vi "caluculate_phase_diff.vi"() -> ()   [LabVIEW 2014]
uses:
  <vilib>/Analysis/3filter.llb/Filter Passband Type.ctl
  <vilib>/addons/Digital Filter Design/_Objects.llb/DFD Quantization Settings.ctl
  <vilib>/addons/Digital Filter Design/_Objects.llb/DFD Quantization Sources.ctl
  <vilib>/measure/matone.llb/Extract Single Tone Information 1 Chan.vi
  <vilib>/Analysis/3filter.llb/IIR Filter (DBL).vi
  <vilib>/addons/Digital Filter Design/Process.llb/DFD Filtering (Array).vi
  <vilib>/addons/Digital Filter Design/FXPLib.llb/DFD FXP to I16 (scalar).vi
  <vilib>/Waveform/WDTOps.llb/WDT Get Waveform Subset DBL.vi
  <vilib>/addons/Digital Filter Design/FXPModel.llb/DFD FXP Quantize Coef (Easy).vi
  <vilib>/addons/Digital Filter Design/CodeGen.llb/DFD FXP C Code Generator.vi
  <vilib>/Utility/VariantDataType/GetNumericFxpInfo.vi
  <vilib>/addons/Digital Filter Design/FXPSim.llb/dfd_Check Input FXP Settings.vi
  <vilib>/addons/Digital Filter Design/FXPSim.llb/dfd_Check SRate Simulation Integer Input.vi
  <vilib>/addons/Digital Filter Design/FXPSim.llb/dfd_FXP Simu.vi
  <vilib>/addons/Digital Filter Design/FXPLib.llb/DFD I16 to FXP (scalar).vi
  <vilib>/addons/Digital Filter Design/_Objects.llb/DFD FXP Statistics Data.ctl
  <vilib>/addons/Digital Filter Design/FXPSim.llb/SimXnode/DFD FXP Simulation.xnode
  <vilib>/addons/Digital Filter Design/_Objects.llb/DFD Filter Obj.ctl
  <vilib>/addons/Digital Filter Design/_Objects.llb/DFD Filter Coef.ctl
  <vilib>/addons/Digital Filter Design/_Objects.llb/DFD Filter Structure Type Selector.ctl
  <vilib>/addons/Digital Filter Design/_Objects.llb/dfd_Internal Quantization Settings.ctl
  <vilib>/addons/Digital Filter Design/_Objects.llb/dfd_Internal Quantization Srcs.ctl
  <vilib>/addons/Digital Filter Design/_Objects.llb/DFD Coef Norm Type.ctl
  <vilib>/measure/NI_MABase.lvlib
  <vilib>/measure/NI_MAPro.lvlib
  <vilib>/Analysis/NI_AALBase.lvlib
  <vilib>/addons/Digital Filter Design/NI_DigFilterLicensed.lvlib
  <vilib>/addons/Digital Filter Design/NI_DigFilter_FXP.lvlib
  <vilib>/Utility/VariantDataType/VariantType.lvlib
panel:
  in  "布尔":bool
  out "difference equation 2":picture
  out "difference equation":picture
  out "denominator":dbl[](array[numeric])
  out "numerator":dbl[](array[numeric])
  in  "filter type":T1(ring)=enum."Bandpass"
  in  "low cutoff freq [Hz]":dbl=40.0
  in  "high cutoff freq [Hz]":dbl=60.0
  in  "order 2":i32=4
  out "x-y 2":dbl
  out "detected frequency":dbl caption="检测到的频率" format="%.2p"
  in  "high cutoff freq: fh":dbl=60.0 format="%#_13g"
  in  "order":i32=3 caption="阶数"
  in  "low cutoff freq: fl":dbl=40.0 caption="低截止频率:fl" format="%0.4f"
  out "x-y":dbl
  out "波形图":waveform(dbl)[](graph)
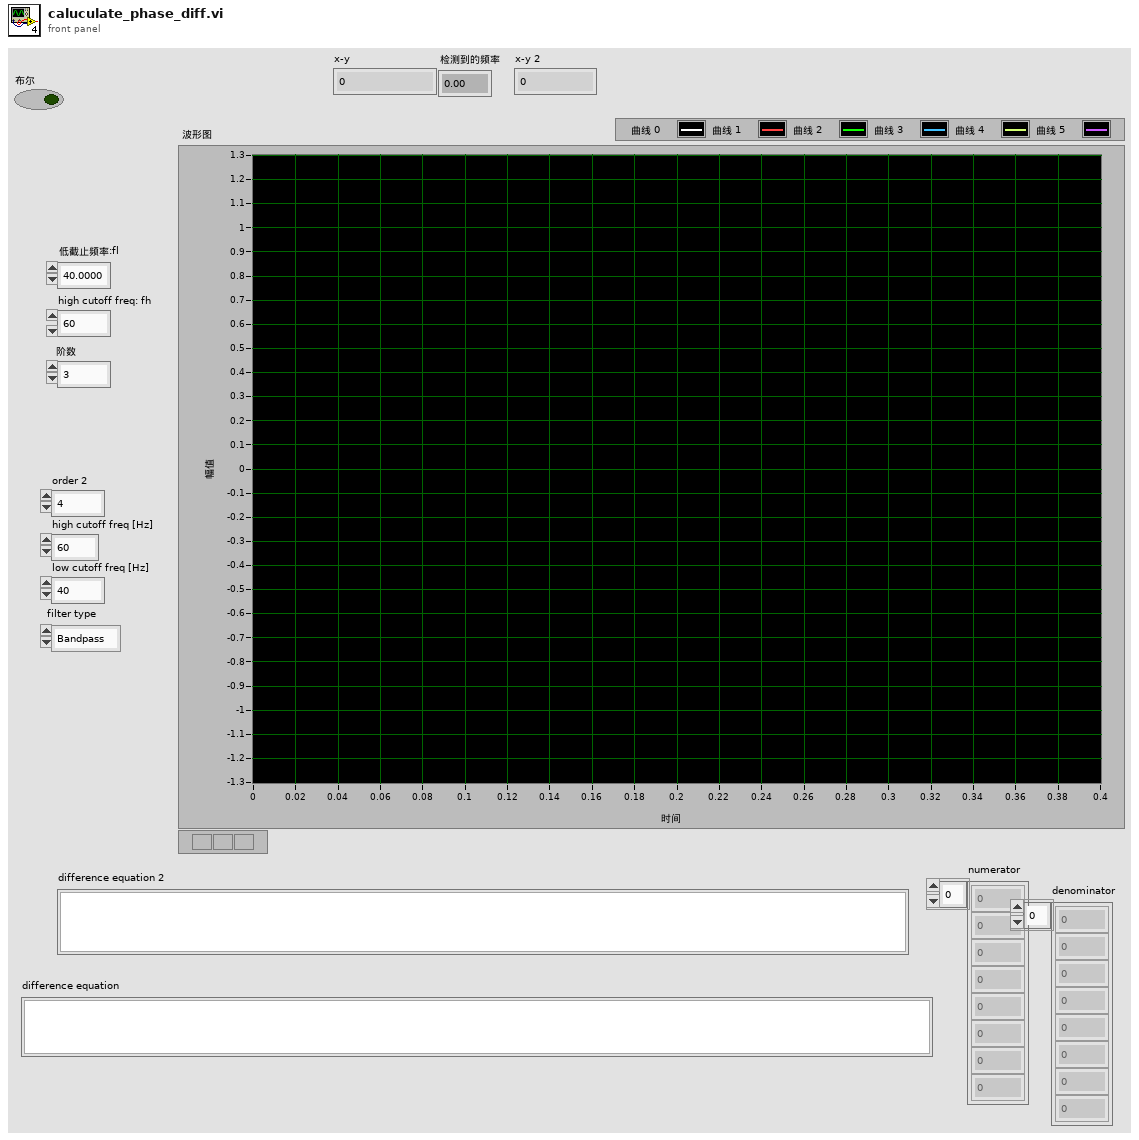
[diagram p1: front panel]
types:
  T1 = enum16{"Lowpass", "Highpass", "Bandpass", "Bandstop"}
  T2 = cluster{"gain processing":u16, "gain word length":i16}
  T3 = typedef "NI_AALBase.lvlib/Filter Passband Type.ctl" = enum32{"Lowpass", "Highpass", "Bandpass", "Bandstop"}
  T4 = cluster{"filter structure":enum32{"IIR 2nd Order", "IIR 4th Order"}, "Reverse Coefficients":dbl[], "Forward Coefficients":dbl[]}
  T5 = typedef "NI_DigFilterLicensed.lvlib/DFD Filter Obj.ctl" = cluster{"mSRate_Fs":dbl, "mSRate_Version":string, "mSRate_Comments":string, "mSRate_OrgCoef":T6, "mSRate_CurCoef":T6, "mSRate_Quantized?":bool, "mSRate_QCoef":T6, "mSRate_QSettings":T8[], "mSRate_Order":i32, "mSRate_Scaling":cluster{"mSRate_ScaleByPowerOf2?":bool, "mSRate_ScaleType":T10}}
  T6 = typedef "NI_DigFilterLicensed.lvlib/DFD Filter Coef.ctl" = cluster{"type":T7, "gain":dbl, "coef a (k)":dbl[], "coef b (v)":dbl[]}
  T7 = typedef "NI_DigFilterLicensed.lvlib/DFD Filter Structure Type Selector.ctl" = enum16{"Undefined", "FIR Direct Form", "FIR Direct Form Transposed", "FIR Symmetric", "FIR Antisymmetric", "IIR Direct Form I", "IIR Direct Form I Transposed", "IIR Direct Form II", "IIR Direct Form II Transposed", "IIR Cascaded Second Order Sections Form I", "IIR Cascaded Second Order Sections Form I Transposed", "IIR Cascaded Second Order Sections Form II", "IIR Cascaded Second Order Sections Form II Transposed", "Lattice Allpass (basic sections)", "Lattice Allpass (one multiplier sections)", "Lattice Allpass (normalized sections)", "Lattice AR (basic sections)", "Lattice AR (one multiplier sections)", "Lattice AR (normalized sections)", "Lattice MA (minimum phase)", "Lattice MA (maximum phase)", "Lattice ARMA (basic sections)", "Lattice ARMA (one multiplier sections)", "Lattice ARMA (normalized sections)"}
  T8 = typedef "NI_DigFilterLicensed.lvlib/dfd_Internal Quantization Settings.ctl" = cluster{"source":T9, "wl":i16, "iwl":i16, "overflow mode":enum16{"Saturation", "Wrap"}, "rounding mode":enum16{"Nearest", "Truncation"}, "signed?":bool}
  T9 = typedef "NI_DigFilterLicensed.lvlib/dfd_Internal Quantization Srcs.ctl" = u16
  T10 = typedef "NI_DigFilterLicensed.lvlib/DFD Coef Norm Type.ctl" = enum16{"No Norm", "Time Domain 1-Norm", "Time Domain 2-Norm", "Time Domain Inf-Norm"}
  T11 = typedef "NI_DigFilterLicensed.lvlib/DFD Quantization Settings.ctl" = cluster{"source":T12, "wl":i16, "iwl":i16, "overflow mode":enum16{"Saturation", "Wrap"}, "rounding mode":enum16{"Nearest", "Truncation"}, "signed?":bool}
  T12 = typedef "NI_DigFilterLicensed.lvlib/DFD Quantization Sources.ctl" = u16
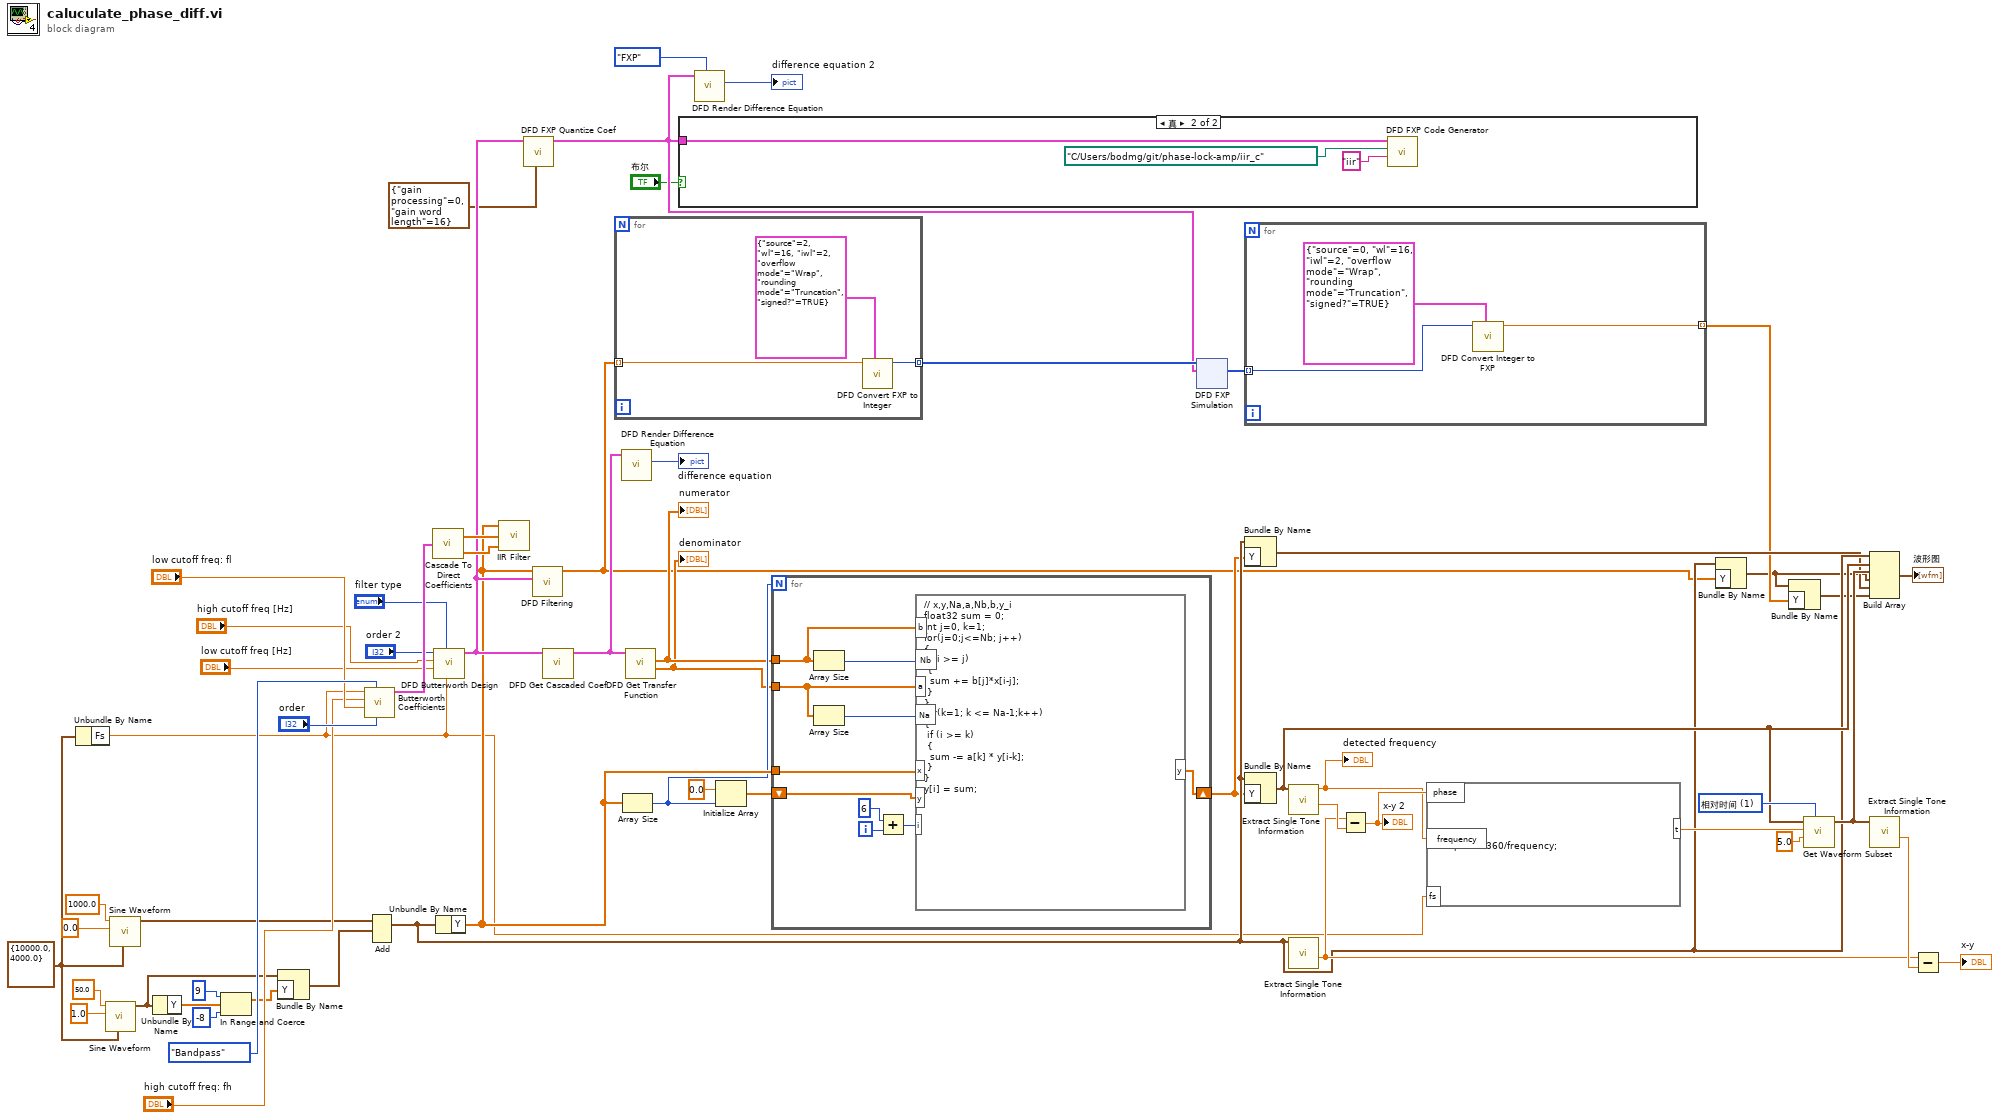
[diagram p0: block diagram]
diagram:
  w46 = u16 1 items=["采样", "相对时间"] ("start/duration format")
  w41 = cluster{"Fs":dbl, "#s":dbl} {"Fs"=10000.0, "#s"=4000.0} ("sampling info")
  n1 = Unbundle By Name(w41) -> ("Fs"=w4:dbl)
  n2 = call <vilib>:"Sine Waveform.vi"("sampling info"=w41, "amplitude"=1.0, "frequency"=50.0) -> ("signal out"=w33:waveform(dbl))  [unwired: 7 in, 1 out]
  n3 = call <vilib>:"Sine Waveform.vi"("sampling info"=w41, "amplitude"=0.0, "frequency"=1000.0) -> ("signal out"=w38:waveform(dbl))  [unwired: 7 in, 1 out]
  n4 = Unbundle By Name(w33) -> ("Y"=w37:dbl[])
  n5 = In Range and Coerce(upper limit=9, x=w37, lower limit=-8) -> (coerced(x)=w34:dbl[])  [unwired: 1 out]
  n6 = Bundle By Name(cluster=w33, "Y"=w34) -> (w32:waveform(dbl))
  n7 = call <vilib>:"Butterworth Coefficients.vi"("order"="order", "filter type"=Filter_Passband_Type."Bandpass", "low cutoff freq: fl"="low cutoff freq: fl", "high cutoff freq: fh"="high cutoff freq: fh", "sampling freq: fs"=w4) -> ("IIR Filter Cluster"=w51:T4)  [unwired: 5 in, 1 out]
  n8 = Add(1:w32, 2:w38) -> (0:w13:waveform(dbl))  [unwired: 1 in, 1 out]
  n9 = call <vilib>:"Cascade To Direct Coefficients.vi"("IIR Filter Cluster"=w51) -> ("Reverse Coefficients"=w29:dbl[], "Forward Coefficients"=w30:dbl[])
  n10 = call <vilib>:"DFD Butterworth Design.vi"("fs [Hz]"=w4, "filter type"="filter type", "low cutoff freq [Hz]"="low cutoff freq [Hz]", "high cutoff freq [Hz]"="high cutoff freq [Hz]", "order"="order 2") -> ("filter out"=w22:T5)  [unwired: 5 in, 1 out]
  n11 = Unbundle By Name(w13) -> ("Y"=w18:dbl[])
  n12 = call-poly <vilib>:"IIR Filter.vi"("Forward Coefficients"=w30, "Reverse Coefficients"=w29, "X"=w18) -> ()  [unwired: 1 in, 2 out]
  n13 = call-poly <vilib>:"DFD FXP Quantize Coef.vi"("gain settings"=T2 {"gain processing"=0, "gain word length"=16}, "filter in"=w22) -> ("filter out"=w3:T5)  [unwired: 8 in, 1 out]
  n14 = call-poly <vilib>:"DFD Filtering.vi"("filter"=w22, "signal in"=w18) -> ("signal out"=w10:dbl[])  [unwired: 8 in, 1 out]
  n15 = call <vilib>:"DFD Get Cascaded Coef.vi"("filter in"=w22) -> ("filter out"=w24:T5)  [unwired: 7 in, 3 out]
  n16 = for {
    tunnel: w10 -> [w62] mode=indexing
    tunnel: [w61] -> w9 mode=indexing
    n17 = call-poly <vilib>:"DFD Convert FXP to Integer.vi"("quantization settings"=T11 {"source"=2, "wl"=16, "iwl"=2, "overflow mode"=enum."Wrap", "rounding mode"=enum."Truncation", "signed?"=TRUE}, "FXP value"=w62) -> ("I16"=w61:i16)  [unwired: 8 in, 1 out]
  }
  n18 = call <vilib>:"DFD Render Difference Equation.vi"("filter in"=w24) -> ("difference equation"=→"difference equation":picture)  [unwired: 7 in, 3 out]
  n19 = Array Size(array=w18) -> (size(s)=w16:i32)
  n20 = call <vilib>:"DFD Get Transfer Function.vi"("filter in"=w24) -> ("denominator"=w14:dbl[], "numerator"=w15:dbl[])  [unwired: 7 in, 2 out]
  "numerator" <- w15
  "denominator" <- w14
  n21 = case shown="真" "布尔" {
    tunnel: w3 -> [_ w65]
    frame False {
    }
    frame True {
      n22 = call-poly <vilib>:"DFD FXP Code Generator.vi"("filter name"="iir", "destination folder"=path "C:/Users/bodmg/git/phase-lock-amp/iir_c", "filter in"=w65) -> ()  [unwired: 7 in, 2 out]
    }
  }
  n23 = call <vilib>:"DFD Render Difference Equation.vi"("type (FLP)"=enum16{"FLP", "FXP"}."FXP", "filter in"=w3) -> ("difference equation"=→"difference equation 2":picture)  [unwired: 6 in, 3 out]
  n24 = Initialize Array(0.0 ("元素"), w16) -> (w17:dbl[])
  n25 = for {
    N: w16 -> [_]
    tunnel: w18 -> [w75]
    shift-right: [w70] -> w11
    shift-left: w17 -> [w74]
    tunnel: w15 -> [w69]
    tunnel: w14 -> [w66]
    i -> [w73]
    n26 = Array Size(array=w69) -> (size(s)=w68:i32)
    n27 = Array Size(array=w66) -> (size(s)=w67:i32)
    n28 = Add(x=6, y=w73) -> (x+y=w72:i32)
    n29 = formula code="// x,y,Na,a,Nb,b,y_i\nfloat32 sum = 0;\nint j=0, k=1;\nfor(j=0;j<=Nb; j++)\n{\n\tif(i >= j)\n\t{\n\t\tsum += b[j]*x[i-j];\n\t}\n}\nfor(k=1; k <= Na-1;k++)\n{\n\tif (i >= k)\n\t{\n\t\tsum -= a[k] * y[i-k];\n\t}\n}\ny[i] = sum;"("b"=w69, "Nb"=w68, "a"=w66, "Na"=w67, "i"=w72, "x"=w75, "y"=w74) -> ("y"=w70:dbl[])
  }
  n30 = xnode "DFD FXP Simulation"("filter in"=w3, "signal in"=w9) -> ("integer signal out"=w8:i32[])  [unwired: 4 in, 3 out]
  n31 = for {
    tunnel: w8 -> [w78] mode=indexing
    tunnel: [w77] -> w7 mode=indexing
    n32 = call-poly <vilib>:"DFD Convert Integer to FXP.vi"("quantization settings"=T11 {"source"=0, "wl"=16, "iwl"=2, "overflow mode"=enum."Wrap", "rounding mode"=enum."Truncation", "signed?"=TRUE}, "I16"=w78) -> ("FXP value"=w77:dbl)  [unwired: 8 in, 1 out]
  }
  n33 = Bundle By Name(cluster=w13, "Y"=w11) -> (w12:waveform(dbl))
  n34 = Bundle By Name(cluster=w13, "Y"=w11) -> (w31:waveform(dbl))
  n35 = call-poly <vilib>:"Extract Single Tone Information.vi"("time signal in"=w31) -> ("detected phase (deg)"=w56:dbl, "detected frequency"=w49:dbl)  [unwired: 5 in, 4 out]
  "detected frequency" <- w49
  n36 = call-poly <vilib>:"Extract Single Tone Information.vi"("time signal in"=w13) -> ("detected phase (deg)"=w44:dbl)  [unwired: 5 in, 5 out]
  n37 = Subtract(x=w44, y=w56) -> (x-y=w50:dbl)
  "x-y 2" <- w50
  n38 = formula code="t = phase/360/frequency;"("phase"=w50, "frequency"=w49, "fs"=w4) -> ("t"=w48:dbl)
  n39 = Bundle By Name(cluster=w13, "Y"=w10) -> (w6:waveform(dbl))
  n40 = Bundle By Name(cluster=w6, "Y"=w7) -> (w5:waveform(dbl))
  n41 = call-poly <vilib>:"Get Waveform Subset.vi"("start/duration format"=w46, "duration"=5.0, "start samples/time"=w48, "waveform in"=w31) -> ("waveform out"=w42:waveform(dbl))  [unwired: 2 in, 3 out]
  n42 = Build Array(w13, w31, w42, w6, w12, w5) -> (→"波形图":waveform(dbl)[])
  n43 = call-poly <vilib>:"Extract Single Tone Information.vi"("time signal in"=w42) -> ("detected phase (deg)"=w45:dbl)  [unwired: 5 in, 5 out]
  n44 = Subtract(x=w44, y=w45) -> (x-y=→"x-y":dbl)
